vi "globals4.vi"() -> ()   [LabVIEW 2011]
uses:
  relaySpec.ctl
panel:
  in  "Global Variables":T1(tab)
  out "GPIB Address":string="23"
  out "Log File Path":path
  out "Byte Stream File Refnum":refnum<file>
  out "Log String":string
  out "Temperature Controller RS232":refnum<visa-resource-name>="COM1"
  out "Begin Time":timestamp
  out "Current Time":timestamp
  out "Seq Step Time (s)":dbl=0.01
  out "Last Step":i32
  out "Log Path":path
  out "Growth Database":path=path "C:/MOCVD/MOCVD_Growths.accdb"
  out "Growth Sequence Preferences":path=path "C:/MOCVD/GrowthSequencePreferences.ini"
  in  "Mass flow controllers":cluster{"MFC Range":u16, "MFC Name":string}[](array[cluster]) {"MFC Range" items=["0-10 sccm", "0-100 sccm", "0-1000 sccm"]}
  in  "Multiprogrammer Card Slots":T2={"Relay Card Slots"={"Card 1"=10, "Card 2"=11, "Card 3"=12, "Card 4"=13, "Card 5"=14}, "Quad D/A Card Slots"={"Card 1"=4, "Card 2"=5, "Card 3"=7, "Card 4"=8, "Card 5"=9, "Card 6 (12-bit)"=9}, "A/D Card Slots"={"Scanner"=0, "High-Speed A/D"=1, "Timer"=2}} {"A/D Card Slots"."Timer" items=["400@", "401A", "402B", "403C", "404D", "405E", "406F", "407G", "408H", "409I", "410J", "411K", "412L", "413M", "414N"]; "A/D Card Slots"."High-Speed A/D" items=["400@", "401A", "402B", "403C", "404D", "405E", "406F", "407G", "408H", "409I", "410J", "411K", "412L", "413M", "414N"]; "A/D Card Slots"."Scanner" items=["400@", "401A", "402B", "403C", "404D", "405E", "406F", "407G", "408H", "409I", "410J", "411K", "412L", "413M", "414N"]; "Quad D/A Card Slots"."Card 6 (12-bit)" items=["400@", "401A", "402B", "403C", "404D", "405E", "406F", "407G", "408H", "409I", "410J", "411K", "412L", "413M", "414N"]; "Quad D/A Card Slots"."Card 1" items=["400@", "401A", "402B", "403C", "404D", "405E", "406F", "407G", "408H", "409I", "410J", "411K", "412L", "413M", "414N"]; "Quad D/A Card Slots"."Card 2" items=["400@", "401A", "402B", "403C", "404D", "405E", "406F", "407G", "408H", "409I", "410J", "411K", "412L", "413M", "414N"]; "Quad D/A Card Slots"."Card 3" items=["400@", "401A", "402B", "403C", "404D", "405E", "406F", "407G", "408H", "409I", "410J", "411K", "412L", "413M", "414N"]; "Quad D/A Card Slots"."Card 4" items=["400@", "401A", "402B", "403C", "404D", "405E", "406F", "407G", "408H", "409I", "410J", "411K", "412L", "413M", "414N"]; "Quad D/A Card Slots"."Card 5" items=["400@", "401A", "402B", "403C", "404D", "405E", "406F", "407G", "408H", "409I", "410J", "411K", "412L", "413M", "414N"]; "Relay Card Slots"."Card 5" items=["400@", "401A", "402B", "403C", "404D", "405E", "406F", "407G", "408H", "409I", "410J", "411K", "412L", "413M", "414N"]; "Relay Card Slots"."Card 4" items=["400@", "401A", "402B", "403C", "404D", "405E", "406F", "407G", "408H", "409I", "410J", "411K", "412L", "413M", "414N"]; "Relay Card Slots"."Card 3" items=["400@", "401A", "402B", "403C", "404D", "405E", "406F", "407G", "408H", "409I", "410J", "411K", "412L", "413M", "414N"]; "Relay Card Slots"."Card 2" items=["400@", "401A", "402B", "403C", "404D", "405E", "406F", "407G", "408H", "409I", "410J", "411K", "412L", "413M", "414N"]; "Relay Card Slots"."Card 1" items=["400@", "401A", "402B", "403C", "404D", "405E", "406F", "407G", "408H", "409I", "410J", "411K", "412L", "413M", "414N"]}
  out "Multiprogrammer Relay Functions":T4={"P Gas"={"Remote"={"Card Index"=2, "Relay Index"=0}, "Active"={"Card Index"=2, "Relay Index"=1}, "Gas In"={"Card Index"=2, "Relay Index"=2}, "H2 Flush"={"Card Index"=2, "Relay Index"=3}, "Run"={"Card Index"=2, "Relay Index"=4}}, "Ga bubbler"={"Remote"={"Card Index"=3, "Relay Index"=0}, "Active"={"Card Index"=3, "Relay Index"=1}, "Bubbler In"={"Card Index"=3, "Relay Index"=2}, "Run"={"Card Index"=3, "Relay Index"=3}, "H2 Dilute"={"Card Index"=3, "Relay Index"=4}}, "In bubbler"={"Remote"={"Card Index"=0, "Relay Index"=7}, "Active"={"Card Index"=0, "Relay Index"=8}, "Bubbler In"={"Card Index"=0, "Relay Index"=9}, "Run"={"Card Index"=0, "Relay Index"=10}}, "Al bubbler"={"Remote"={"Card Index"=0, "Relay Index"=3}, "Active"={"Card Index"=0, "Relay Index"=4}, "Bubbler In"={"Card Index"=0, "Relay Index"=5}, "Run"={"Card Index"=0, "Relay Index"=6}}, "As Gas"={"Remote"={"Card Index"=2, "Relay Index"=5}, "Active"={"Card Index"=2, "Relay Index"=6}, "Gas In"={"Card Index"=2, "Relay Index"=7}, "H2 Flush"={"Card Index"=2, "Relay Index"=8}, "Run"={"Card Index"=2, "Relay Index"=9}}, "H2/N2"={"Remote"={"Card Index"=0, "Relay Index"=3}, "H2 On"={"Card Index"=0, "Relay Index"=4}, "N2 On"={"Card Index"=0, "Relay Index"=5}, "Output"={"Card Index"=0, "Relay Index"=6}}} {"H2/N2"."Output"."Card Index" items=["1", "2", "3", "4", "5"]; "H2/N2"."Output"."Relay Index" items=["1", "2", "3", "4", "5", "6", "7", "8", "9", "10", "11", "12"]; "H2/N2"."N2 On"."Card Index" items=["1", "2", "3", "4", "5"]; "H2/N2"."N2 On"."Relay Index" items=["1", "2", "3", "4", "5", "6", "7", "8", "9", "10", "11", "12"]; "H2/N2"."H2 On"."Card Index" items=["1", "2", "3", "4", "5"]; "H2/N2"."H2 On"."Relay Index" items=["1", "2", "3", "4", "5", "6", "7", "8", "9", "10", "11", "12"]; "H2/N2"."Remote"."Card Index" items=["1", "2", "3", "4", "5"]; "H2/N2"."Remote"."Relay Index" items=["1", "2", "3", "4", "5", "6", "7", "8", "9", "10", "11", "12"]; "As Gas"."Run"."Card Index" items=["1", "2", "3", "4", "5"]; "As Gas"."Run"."Relay Index" items=["1", "2", "3", "4", "5", "6", "7", "8", "9", "10", "11", "12"]; "As Gas"."H2 Flush"."Card Index" items=["1", "2", "3", "4", "5"]; "As Gas"."H2 Flush"."Relay Index" items=["1", "2", "3", "4", "5", "6", "7", "8", "9", "10", "11", "12"]; "As Gas"."Gas In"."Card Index" items=["1", "2", "3", "4", "5"]; "As Gas"."Gas In"."Relay Index" items=["1", "2", "3", "4", "5", "6", "7", "8", "9", "10", "11", "12"]; "As Gas"."Active"."Card Index" items=["1", "2", "3", "4", "5"]; "As Gas"."Active"."Relay Index" items=["1", "2", "3", "4", "5", "6", "7", "8", "9", "10", "11", "12"]; "As Gas"."Remote"."Card Index" items=["1", "2", "3", "4", "5"]; "As Gas"."Remote"."Relay Index" items=["1", "2", "3", "4", "5", "6", "7", "8", "9", "10", "11", "12"]; "Al bubbler"."Run"."Card Index" items=["1", "2", "3", "4", "5"]; "Al bubbler"."Run"."Relay Index" items=["1", "2", "3", "4", "5", "6", "7", "8", "9", "10", "11", "12"]; "Al bubbler"."Bubbler In"."Card Index" items=["1", "2", "3", "4", "5"]; "Al bubbler"."Bubbler In"."Relay Index" items=["1", "2", "3", "4", "5", "6", "7", "8", "9", "10", "11", "12"]; "Al bubbler"."Active"."Card Index" items=["1", "2", "3", "4", "5"]; "Al bubbler"."Active"."Relay Index" items=["1", "2", "3", "4", "5", "6", "7", "8", "9", "10", "11", "12"]; "Al bubbler"."Remote"."Card Index" items=["1", "2", "3", "4", "5"]; "Al bubbler"."Remote"."Relay Index" items=["1", "2", "3", "4", "5", "6", "7", "8", "9", "10", "11", "12"]; "In bubbler"."Run"."Card Index" items=["1", "2", "3", "4", "5"]; "In bubbler"."Run"."Relay Index" items=["1", "2", "3", "4", "5", "6", "7", "8", "9", "10", "11", "12"]; "In bubbler"."Bubbler In"."Card Index" items=["1", "2", "3", "4", "5"]; "In bubbler"."Bubbler In"."Relay Index" items=["1", "2", "3", "4", "5", "6", "7", "8", "9", "10", "11", "12"]; "In bubbler"."Active"."Card Index" items=["1", "2", "3", "4", "5"]; "In bubbler"."Active"."Relay Index" items=["1", "2", "3", "4", "5", "6", "7", "8", "9", "10", "11", "12"]; "In bubbler"."Remote"."Card Index" items=["1", "2", "3", "4", "5"]; "In bubbler"."Remote"."Relay Index" items=["1", "2", "3", "4", "5", "6", "7", "8", "9", "10", "11", "12"]; "Ga bubbler"."H2 Dilute"."Card Index" items=["1", "2", "3", "4", "5"]; "Ga bubbler"."H2 Dilute"."Relay Index" items=["1", "2", "3", "4", "5", "6", "7", "8", "9", "10", "11", "12"]; "Ga bubbler"."Run"."Card Index" items=["1", "2", "3", "4", "5"]; "Ga bubbler"."Run"."Relay Index" items=["1", "2", "3", "4", "5", "6", "7", "8", "9", "10", "11", "12"]; "Ga bubbler"."Bubbler In"."Card Index" items=["1", "2", "3", "4", "5"]; "Ga bubbler"."Bubbler In"."Relay Index" items=["1", "2", "3", "4", "5", "6", "7", "8", "9", "10", "11", "12"]; "Ga bubbler"."Active"."Card Index" items=["1", "2", "3", "4", "5"]; "Ga bubbler"."Active"."Relay Index" items=["1", "2", "3", "4", "5", "6", "7", "8", "9", "10", "11", "12"]; "Ga bubbler"."Remote"."Card Index" items=["1", "2", "3", "4", "5"]; "Ga bubbler"."Remote"."Relay Index" items=["1", "2", "3", "4", "5", "6", "7", "8", "9", "10", "11", "12"]; "P Gas"."Run"."Card Index" items=["1", "2", "3", "4", "5"]; "P Gas"."Run"."Relay Index" items=["1", "2", "3", "4", "5", "6", "7", "8", "9", "10", "11", "12"]; "P Gas"."H2 Flush"."Card Index" items=["1", "2", "3", "4", "5"]; "P Gas"."H2 Flush"."Relay Index" items=["1", "2", "3", "4", "5", "6", "7", "8", "9", "10", "11", "12"]; "P Gas"."Gas In"."Card Index" items=["1", "2", "3", "4", "5"]; "P Gas"."Gas In"."Relay Index" items=["1", "2", "3", "4", "5", "6", "7", "8", "9", "10", "11", "12"]; "P Gas"."Active"."Card Index" items=["1", "2", "3", "4", "5"]; "P Gas"."Active"."Relay Index" items=["1", "2", "3", "4", "5", "6", "7", "8", "9", "10", "11", "12"]; "P Gas"."Remote"."Card Index" items=["1", "2", "3", "4", "5"]; "P Gas"."Remote"."Relay Index" items=["1", "2", "3", "4", "5", "6", "7", "8", "9", "10", "11", "12"]}
  in  "D/A Cards":T5 {"Single-channel D/A (12-bit) Cards"."Channel 1" items=["N2 flow (NMFC1)", "H2 flow (HMFC1)", "Al2 flow (ALMFC1)", "Ga flow 1 (GAMFC1)", "Ga flow 2 (GAMFC2)", "Ga flow 3 (GAMFC3)", "In flow (INMFC1)", "P bubbler (PLMFC1)", "Plasma feed (ASLMFC1)", "P gas (PGMFC1)", "As gas (ASGMFC1)", "p-dopant flow 1 (PDOPMFC1)", "p-dopant flow 2 (PDOPMFC2)", "p-dopant flow 3 (PDOPMFC3)", "n-dopant flow 1 (NDOPMFC1)", "n-dopant flow 2 (NDOPMFC2)", "n-dopant flow 3 (PDOPMFC3)", "bad", "Fe flow 1 (FEMFC1)", "Fe flow 2 (FEMFC2)", "Fe flow 3 (FEMFC3)"]; "Quad D/A (10-bit) Cards"."Channel 4" items=["N2 flow (NMFC1)", "H2 flow (HMFC1)", "Al2 flow (ALMFC1)", "Ga flow 1 (GAMFC1)", "Ga flow 2 (GAMFC2)", "Ga flow 3 (GAMFC3)", "In flow (INMFC1)", "P bubbler (PLMFC1)", "Plasma feed (ASLMFC1)", "P gas (PGMFC1)", "As gas (ASGMFC1)", "p-dopant flow 1 (PDOPMFC1)", "p-dopant flow 2 (PDOPMFC2)", "p-dopant flow 3 (PDOPMFC3)", "n-dopant flow 1 (NDOPMFC1)", "n-dopant flow 2 (NDOPMFC2)", "n-dopant flow 3 (PDOPMFC3)", "bad", "Fe flow 1 (FEMFC1)", "Fe flow 2 (FEMFC2)", "Fe flow 3 (FEMFC3)"]; "Quad D/A (10-bit) Cards"."Channel 3" items=["N2 flow (NMFC1)", "H2 flow (HMFC1)", "Al2 flow (ALMFC1)", "Ga flow 1 (GAMFC1)", "Ga flow 2 (GAMFC2)", "Ga flow 3 (GAMFC3)", "In flow (INMFC1)", "P bubbler (PLMFC1)", "Plasma feed (ASLMFC1)", "P gas (PGMFC1)", "As gas (ASGMFC1)", "p-dopant flow 1 (PDOPMFC1)", "p-dopant flow 2 (PDOPMFC2)", "p-dopant flow 3 (PDOPMFC3)", "n-dopant flow 1 (NDOPMFC1)", "n-dopant flow 2 (NDOPMFC2)", "n-dopant flow 3 (PDOPMFC3)", "bad", "Fe flow 1 (FEMFC1)", "Fe flow 2 (FEMFC2)", "Fe flow 3 (FEMFC3)"]; "Quad D/A (10-bit) Cards"."Channel 2" items=["N2 flow (NMFC1)", "H2 flow (HMFC1)", "Al2 flow (ALMFC1)", "Ga flow 1 (GAMFC1)", "Ga flow 2 (GAMFC2)", "Ga flow 3 (GAMFC3)", "In flow (INMFC1)", "P bubbler (PLMFC1)", "Plasma feed (ASLMFC1)", "P gas (PGMFC1)", "As gas (ASGMFC1)", "p-dopant flow 1 (PDOPMFC1)", "p-dopant flow 2 (PDOPMFC2)", "p-dopant flow 3 (PDOPMFC3)", "n-dopant flow 1 (NDOPMFC1)", "n-dopant flow 2 (NDOPMFC2)", "n-dopant flow 3 (PDOPMFC3)", "bad", "Fe flow 1 (FEMFC1)", "Fe flow 2 (FEMFC2)", "Fe flow 3 (FEMFC3)"]; "Quad D/A (10-bit) Cards"."Channel 1" items=["N2 flow (NMFC1)", "H2 flow (HMFC1)", "Al2 flow (ALMFC1)", "Ga flow 1 (GAMFC1)", "Ga flow 2 (GAMFC2)", "Ga flow 3 (GAMFC3)", "In flow (INMFC1)", "P bubbler (PLMFC1)", "Plasma feed (ASLMFC1)", "P gas (PGMFC1)", "As gas (ASGMFC1)", "p-dopant flow 1 (PDOPMFC1)", "p-dopant flow 2 (PDOPMFC2)", "p-dopant flow 3 (PDOPMFC3)", "n-dopant flow 1 (NDOPMFC1)", "n-dopant flow 2 (NDOPMFC2)", "n-dopant flow 3 (PDOPMFC3)", "bad", "Fe flow 1 (FEMFC1)", "Fe flow 2 (FEMFC2)", "Fe flow 3 (FEMFC3)"]}
  # "Relay Card #"
  # "Relay #"
  # "Relay Card #"
  # "Relay Card #"
  # "Relay #"
  # "Relay #"
  # "Relay Card #"
  # "Relay #"
  # "Relay #"
  # "Relay Card #"
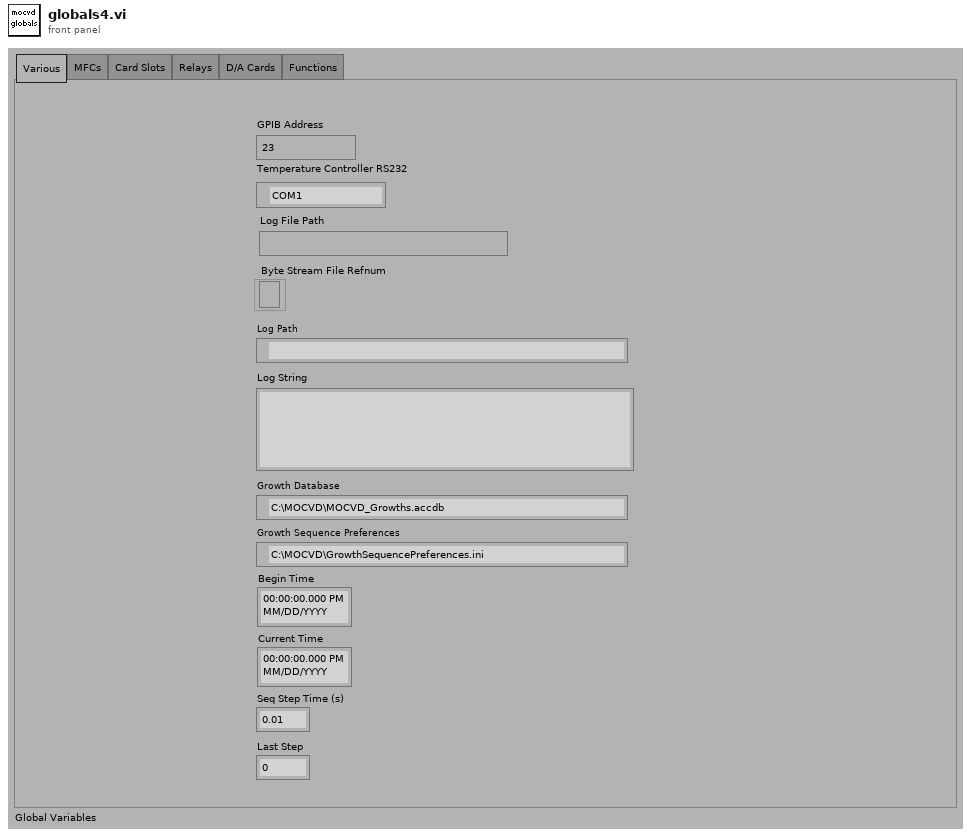
[diagram p1: front panel]
types:
  T1 = enum32{"Various", "MFCs", "Card Slots", "Relays", "D/A Cards", "Functions"}
  T2 = cluster{"Relay Card Slots":cluster{"Card 1":u16, "Card 2":u16, "Card 3":u16, "Card 4":u16, "Card 5":u16}, "Quad D/A Card Slots":cluster{"Card 1":u16, "Card 2":u16, "Card 3":u16, "Card 4":u16, "Card 5":u16, "Card 6 (12-bit)":u16}, "A/D Card Slots":cluster{"Scanner":u16, "High-Speed A/D":u16, "Timer":u16}}
  T3 = typedef "relaySpec.ctl" = cluster{"Card Index":u16, "Relay Index":u16}
  T4 = cluster{"P Gas":cluster{"Remote":T3, "Active":T3, "Gas In":T3, "H2 Flush":T3, "Run":T3}, "Ga bubbler":cluster{"Remote":T3, "Active":T3, "Bubbler In":T3, "Run":T3, "H2 Dilute":T3}, "In bubbler":cluster{"Remote":T3, "Active":T3, "Bubbler In":T3, "Run":T3}, "Al bubbler":cluster{"Remote":T3, "Active":T3, "Bubbler In":T3, "Run":T3}, "As Gas":cluster{"Remote":T3, "Active":T3, "Gas In":T3, "H2 Flush":T3, "Run":T3}, "H2/N2":cluster{"Remote":T3, "H2 On":T3, "N2 On":T3, "Output":T3}}
  T5 = cluster{"Quad D/A (10-bit) Cards":cluster{"Channel 1":u16, "Channel 2":u16, "Channel 3":u16, "Channel 4":u16, "Name":string}[], "Single-channel D/A (12-bit) Cards":cluster{"Name":string, "Channel 1":u16}[]}
diagram:
